vi "Error Message.vi"(8 "error in (no error)":errorcluster, 10 "Type of Dialog (OK msg:1)":i32(ring)=1 items=["no dialog", "OK message", "continue or stop message"], 11 "VISA resource name":refnum<visa-resource-name>) -> (0 "error out":errorcluster, 1 "Error Message (empty)":string, 2 "Error Code (0)":i32, 3 "VISA resource name out":refnum<visa-resource-name>, 7 "status":bool)   [LabVIEW 2016, in "Agilent 428X Series.lvlib"]
doc: "This VI contains all the intrument specific error codes and descriptions. Use this VI after executing several instrument driver VIs to recognize and display any errors that may have occurred."
uses:
  <instrlib>/Agilent 428X Series/Agilent 428X Series.lvlib
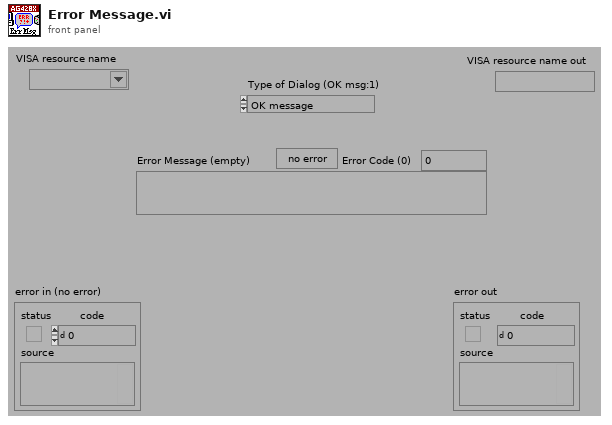
[diagram p1: front panel]
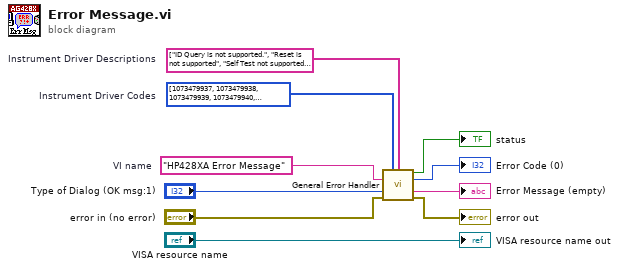
[diagram p0: block diagram]
diagram:
  w2 = i32[] [1073479937, 1073479938, 1073479939, 1073479940, 1073479941]  # Instrument Driver Codes
  w1 = string[] ["ID Query is not supported.", "Reset is not supported", "Self Test not supported.", "Error Query not supported.", "Revision Query not supported."]  # Instrument Driver Descriptions
  w7 = "HP428XA Error Message"  # VI name
  n1 = call <vilib>:"General Error Handler.vi"("[user-defined codes]"=w2, "[user-defined descriptions]"=w1, "[error source] (\" \")"=w7, "type of dialog (OK msg:1)"="Type of Dialog (OK msg:1)", "error in (no error)"="error in (no error)") -> ("error?"=→"status":bool, "code out"=→"Error Code (0)":i32, "message"=→"Error Message (empty)":string, "error out"=→"error out":errorcluster)  [unwired: 6 in, 1 out]
  "VISA resource name out" <- "VISA resource name"
